vi "GetLogString.vi"(8 "error":errorcluster, 11 "VISA resource":refnum<visa-resource-name>) -> (0 "error out":errorcluster, 1 "log entry string":string, 3 "VISA resource out":refnum<visa-resource-name>)   [LabVIEW 2023, in "BigSkyControl.lvlib"]
uses:
  BigSkyControl.lvlib
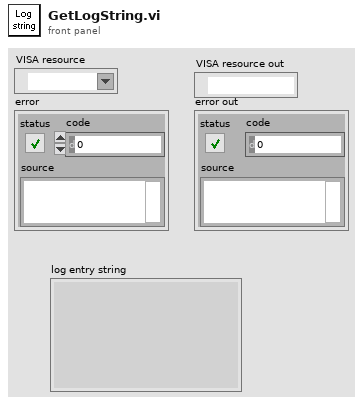
[diagram p1: front panel]
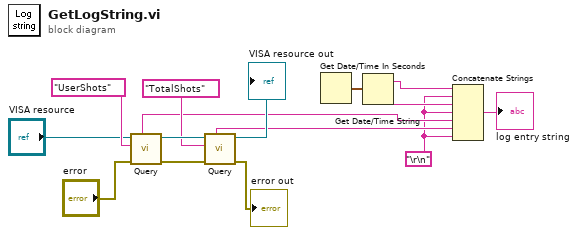
[diagram p0: block diagram]
diagram:
  w2 = "\r\n"
  n1 = call "Query.vi"("error"="error", "Quantity"="UserShots", "VISA resource name"="VISA resource") -> ("error out"=w9:errorcluster, "VISA resource name out"=w11:refnum<visa-resource-name>, "Response"=w4:string)  [unwired: 3 in, 1 out]
  n2 = call "Query.vi"("error"=w9, "Quantity"="TotalShots", "VISA resource name"=w11) -> ("error out"=→"error out":errorcluster, "VISA resource name out"=→"VISA resource out":refnum<visa-resource-name>, "Response"=w5:string)  [unwired: 3 in, 1 out]
  n3 = Get Date/Time In Seconds() -> (seconds since 1Jan1904=w14:timestamp)
  n4 = Get Date/Time String(seconds (now)=w14) -> (date string=w15:string, time string=w3:string)  [unwired: 2 in]
  n5 = Concatenate Strings(w15, w2, w3, w2, w4, w5, w2) -> (→"log entry string":string)
